vi "simulation Control Init.vi"(8 "error in (no error)":errorcluster) -> (0 "error out":errorcluster)   [LabVIEW 2019, in "libSimulationControl.lvlib"]
doc: "void simulationControlInit();"
uses:
  libSimulationControl.lvlib
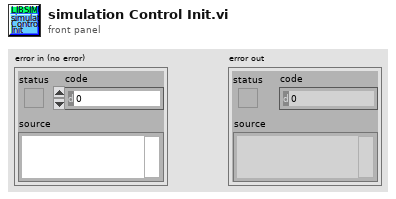
[diagram p1: front panel]
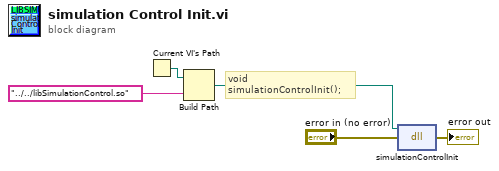
[diagram p0: block diagram]
diagram:
  # "void simulationControlInit();"
  n1 = Current VI's Path() -> (path=w3:path)
  n2 = Build Path(base path=w3, name or relative path="../../libSimulationControl.so") -> (appended path=w1:path)
  n3 = dll-call lib="home/paul/Schreibtisch/Biogas_plant_setup/LabView/lib/libSimulationControl/libSimulationControl.*" fn="simulationControlInit"(path in=w1, error in="error in (no error)") -> (error out=→"error out":errorcluster)  [unwired: 2 in, 1 out]
